vi "Joystick Adjustment to Drive Straight.vi"() -> ()   [LabVIEW 2017]
panel:
  out "Right Motor Value":dbl
  out "Left Motor Value":dbl
  in  "Turning Joystick Input":dbl
  in  "Speed Joystick Input":dbl
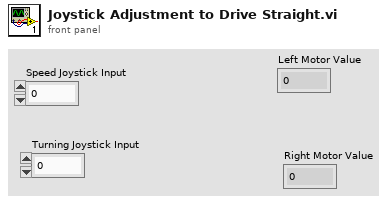
[diagram p1: front panel]
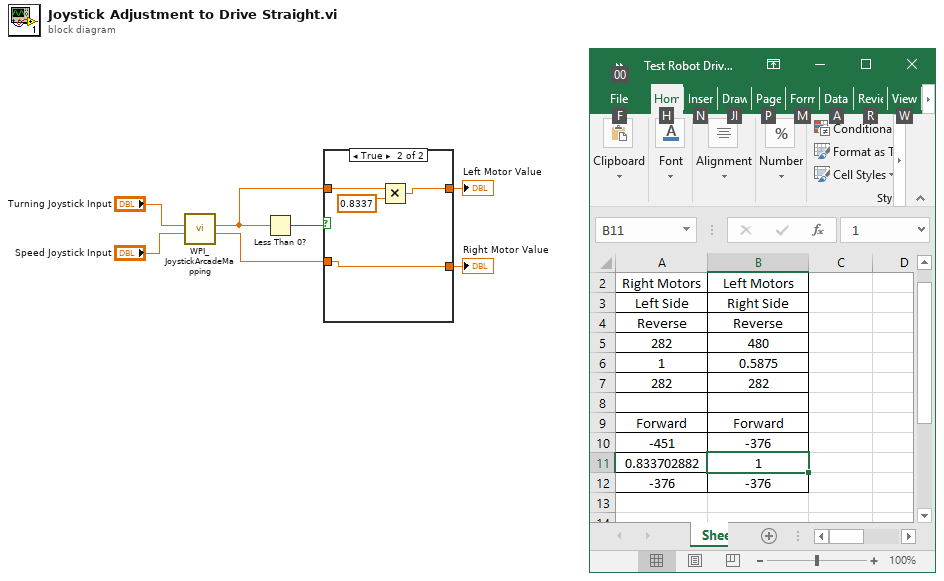
[diagram p0: block diagram]
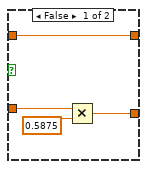
[diagram p2: hidden frame]
diagram:
  n1 = call <vilib>:"WPI_JoystickArcadeMapping.vi"("Y axis value"="Speed Joystick Input", "X axis value"="Turning Joystick Input") -> ("Right Motor Value"=w3:dbl, "Left Motor Value"=w4:dbl)  [unwired: 8 in]
  n2 = Less Than 0?(x=w4) -> (x < 0?=w5:bool)
  n3 = case shown="True" w5 {
    tunnel: [w11 w14] -> w2
    tunnel: w4 -> [w11 w15]
    tunnel: w3 -> [w10 w12]
    tunnel: [w8 w12] -> w1
    frame False {
      n4 = Multiply(x=w10, y=0.5875) -> (x*y=w8:dbl)
    }
    frame True {
      n5 = Multiply(x=w15, y=0.8337) -> (x*y=w14:dbl)
    }
  }
  "Left Motor Value" <- w2
  "Right Motor Value" <- w1
